vi "Test Record.vi"() -> ()   [LabVIEW 2017]
uses:
  src/Record.Error/Record.Error.lvclass
  \\192.168.1.40\Neosoft/Partage/Dossiers Personnels/BRO/DevTools_BR/wc/ErrorLog/src/Record/Record.lvclass
  src/Record/Record.lvclass
panel:
  out "Record String":string
  out "Record.Error String":string
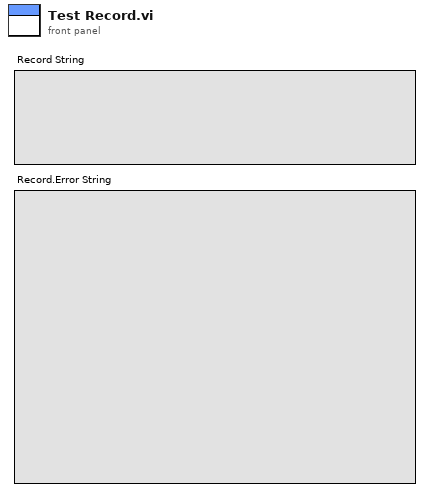
[diagram p1: front panel]
types:
  T1 = enum16{"DEBUG", "INFO", "WARNING", "ERROR", "CRITICAL"}
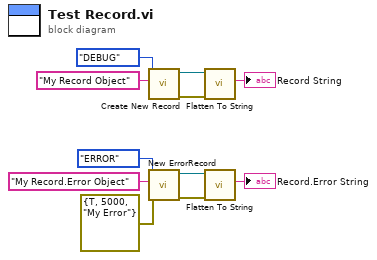
[diagram p0: block diagram]
diagram:
  n1 = call "Create New Record.vi"("Message"="My Record Object", "Level"=T1."DEBUG") -> ("error out"=w7:errorcluster, "Record out"=w8:refnum<class "Record.lvclass">)  [unwired: 8 in]
  n2 = call "New ErrorRecord.vi"("Error"=errorcluster {"status"=TRUE, "code"=5000, "source"="My Error"}, "Message"="My Record.Error Object", "Level"=T1."ERROR") -> ("error out"=w3:errorcluster, "Record.Error out"=w11:refnum<class "Record.Error.lvclass">)  [unwired: 7 in]
  n3 = call "Flatten To String.vi"("error in (no error)"=w7, "Record in"=w8) -> ("String"=→"Record String":string)  [unwired: 7 in, 2 out]
  n4 = call "Flatten To String.vi"("error in (no error)"=w3, "Record in"=w11) -> ("String"=→"Record.Error String":string)  [unwired: 7 in, 2 out]
